vi "UI SaveAs Config.vi"(8 "error in (no error)":errorcluster, 11 "CallActorCenter in":refnum<class "CallActorCenter.lvclass">) -> (0 "error out":errorcluster, 3 "CallActorCenter out":refnum<class "CallActorCenter.lvclass">)   [LabVIEW 2021, in "CallActorCenter.lvclass"]
uses:
  CallActorCenter.lvclass
  CallActorCenter.lvclass/CallActorCenter.ctl
  <userlib>/John_Lib/AbstractActorTemplate/AbstractActorTemplate/UIActorTop.lvclass
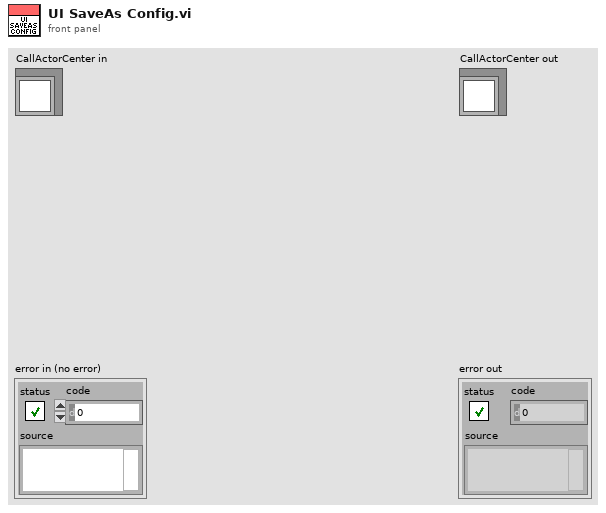
[diagram p1: front panel]
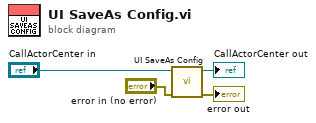
[diagram p0: block diagram]
diagram:
  n1 = call-parent "UI SaveAs Config.vi"("error in (no error)"="error in (no error)", "UIActorTop in"="CallActorCenter in") -> ("error out"=→"error out":errorcluster, "UIActorTop out"=→"CallActorCenter out":refnum<class "CallActorCenter.lvclass">)  [unwired: 8 in]
